vi "Update Multiplication Result Ref.vi"(8 "error in (no error)":errorcluster, 10 "Multiplication Result":dbl, 11 "Calculator Actor in":refnum<class "Calculator Actor.lvclass">) -> (0 "error out":errorcluster, 3 "Calculator Actor out":refnum<class "Calculator Actor.lvclass">)   [LabVIEW 2015, in "Calculator Actor.lvclass"]
uses:
  Calculator Actor.lvclass
  Calculator Actor.lvclass/Calculator Actor.ctl
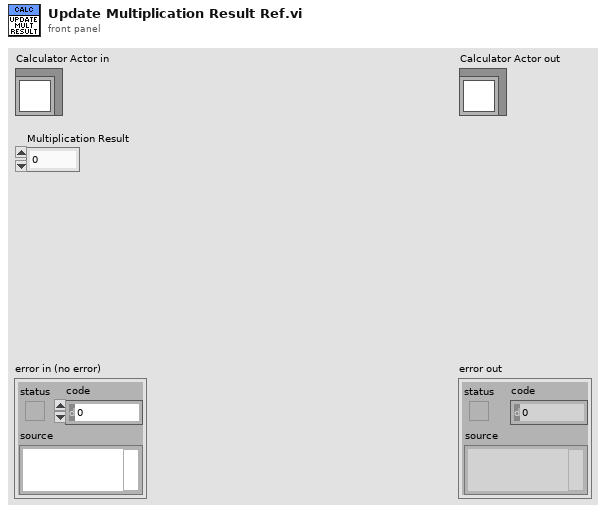
[diagram p1: front panel]
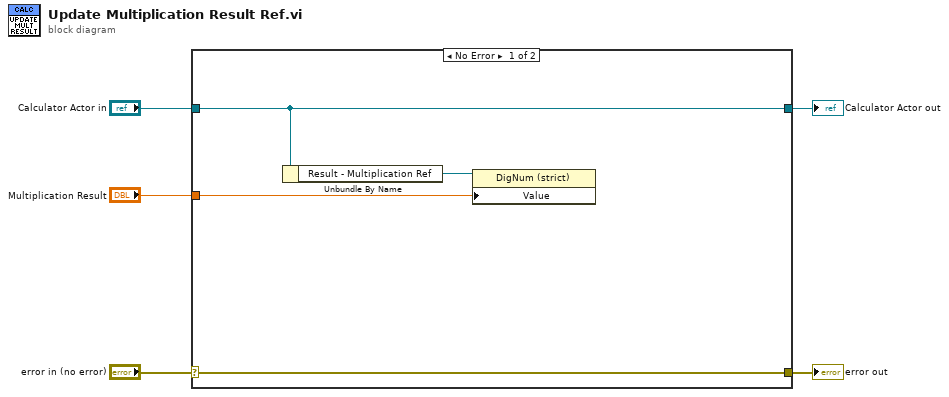
[diagram p0: block diagram]
diagram:
  n1 = case shown="No Error" "error in (no error)" {
    selector: "error in (no error)" -> [w9 w11]
    tunnel: [w9 w11] -> w4
    tunnel: [w8 w10] -> w2
    tunnel: "Calculator Actor in" -> [w8 w10]
    tunnel: "Multiplication Result" -> [w6 _]
    frame No Error {
      n2 = Unbundle By Name(w8) -> ("Result - Multiplication Ref"=w7:refnum<vi>)
      n3 = property class="DigNum (strict)"(reference=w7, "Value"=w6) -> ()  [unwired: 1 in, 2 out]
    }
    frame Error {
    }
  }
  "error out" <- w4
  "Calculator Actor out" <- w2
